vi "List Grouped Tags.vi"(8 "error in (no error)":errorcluster, 11 "Group":string) -> (0 "error out":errorcluster, 1 "Tags Out":string[](array[string]))   [LabVIEW 2010, in "Current Value Table.lvlib"]
doc: "This VI will read an entire group as defined during tag creation or by the FormGroup VI. This VI functions as both the normal and static versions of the group read, as the small performance drop from the group name check is insignificant for reasonably sized groups."
uses:
  Current Value Table.lvlib
  FGVs/Group Memory Methods.ctl
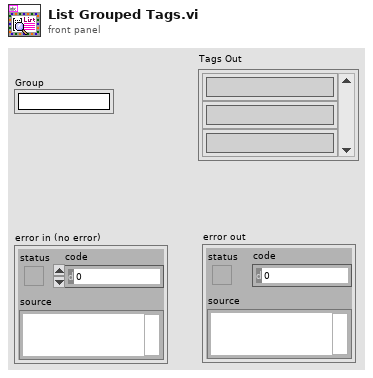
[diagram p1: front panel]
types:
  T1 = typedef "Current Value Table.lvlib/Group Memory Methods.ctl" = enum16{"Clear", "Read Indices in Group", "List Groups", "List Tags by Type", "List Tags", "Delete Group", "Check Group Existence", "Create Group"}
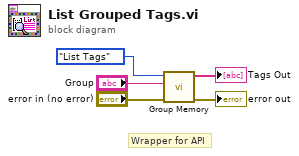
[diagram p0: block diagram]
diagram:
  # "Wrapper for API"
  n1 = call "Group Memory.vi"("error in (no error)"="error in (no error)", "Group"="Group", "Method"=Group_Memory_Methods."List Tags") -> ("error out"=→"error out":errorcluster, "Tags/Groups Out"=→"Tags Out":string[])  [unwired: 5 in, 2 out]
